vi "Test Bench v22 - TDMS.vi"() -> ()   [LabVIEW 2022 SP3]
doc: "Use this template to build a producer/consumer design pattern. Use this template when you need to execute a process, such as data analysis, when a data source, such as a triggered acquisition, produces data at an uneven rate and you need to execute the process when the data becomes available."
uses:
  WhiteNoise.ctl
  <vilib>/Utility/error.llb/DialogType.ctl
  <vilib>/Platform/TimedLoop/XDataNode/timing_clust.ctl
  <vilib>/Platform/TimedLoop/XDataNode/nitl_modes.ctl
  <vilib>/Platform/TimedLoop/XDataNode/wakeup.ctl
  <vilib>/DAQmx/write.llb/DAQmx Write (Analog Wfm 1Chan NSamp).vi
  <vilib>/DAQmx/read.llb/DAQmx Read (Analog Wfm 1Chan NSamp).vi
  <vilib>/DAQmx/miscellaneous.llb/DAQmx Fill In Error Info.vi
  <vilib>/measure/maspectr.llb/FFT Spectrum (Mag-Phase) for 1 Chan.vi
  <vilib>/platform/TimedLoop/XDataNode/XDataNode.xnode
  <vilib>/Platform/TimedLoop/XDataNode/XDNodeRunTimeDep.lvlib
  <vilib>/measure/NI_MAPro.lvlib
panel:
  out "SignalOut":waveform(dbl)(graph)
  out "FFT - Magnitude 2":cluster{"f0":dbl, "df":dbl, "magnitude":dbl[]}(graph)
  in  "view 2":T1={"dB On (F)"=FALSE, "unwrap phase (F)"=TRUE, "convert to degree (F)"=TRUE}
  out "FFT - Phase 2":cluster{"f0":dbl, "df":dbl, "phase":dbl[]}(graph)
  out "Accel":waveform(dbl)(graph)
  out "error out":errorcluster
  in  "stop":bool
  out "Iteration Duration 3":i64
  in  "samples per channel":i32=41200
  in  "Folder to save file to":path=path "C:/Users/LAV-UFSC-2023/Documents/LAV-TCC/Dados-Experimentos/Dados-Bancada-LABVIEW"
  out "# pending insert":i32
  out "# pending remove":i32
  out "# elements in queue":i32
  out "Processor 2":i32=-2
  out "Iteration Duration":i64
  out "Processor":i32=-2
  out "New file path":path
  in  "Log Data":bool=TRUE
  out "Iteration Duration 2":i64
  in  "Enable Output":bool=TRUE
  in  "Signal Output\nControl":enum32{"White Noise", "Harmonic"}(tab)
  in  "White Noise\nParameters":T3={"Seed"=0.0, "Standard Deviation"=2.0, "Reset"=FALSE, "Iterator"=1.0, "Lower Cut-Off"=5.0, "Upper Cut-Off"=350.0} {"Upper Cut-Off" min=5.0 max=350.0 step=10.0; "Lower Cut-Off" min=5.0 max=350.0 step=10.0; "Standard Deviation" min=0.001 max=3.0 step=0.05 format="%0.2p"}
  in  "Hamonic\nParameters":T4={"Waveform Type"=0, "Frequency (Hz)"=10.0, "Amplitude"=0.25} {"Frequency (Hz)" min=5.0 max=350.0 step=10.0 format="%0.2p"; "Waveform Type" items=["Sine Wave", "Triangle Wave", "Square Wave", "Sawtooth Wave"]; "Amplitude" min=0.001 max=0.3 step=0.05 format="%0.2p"}
  # "Debug Pannel"
  # "Filter"
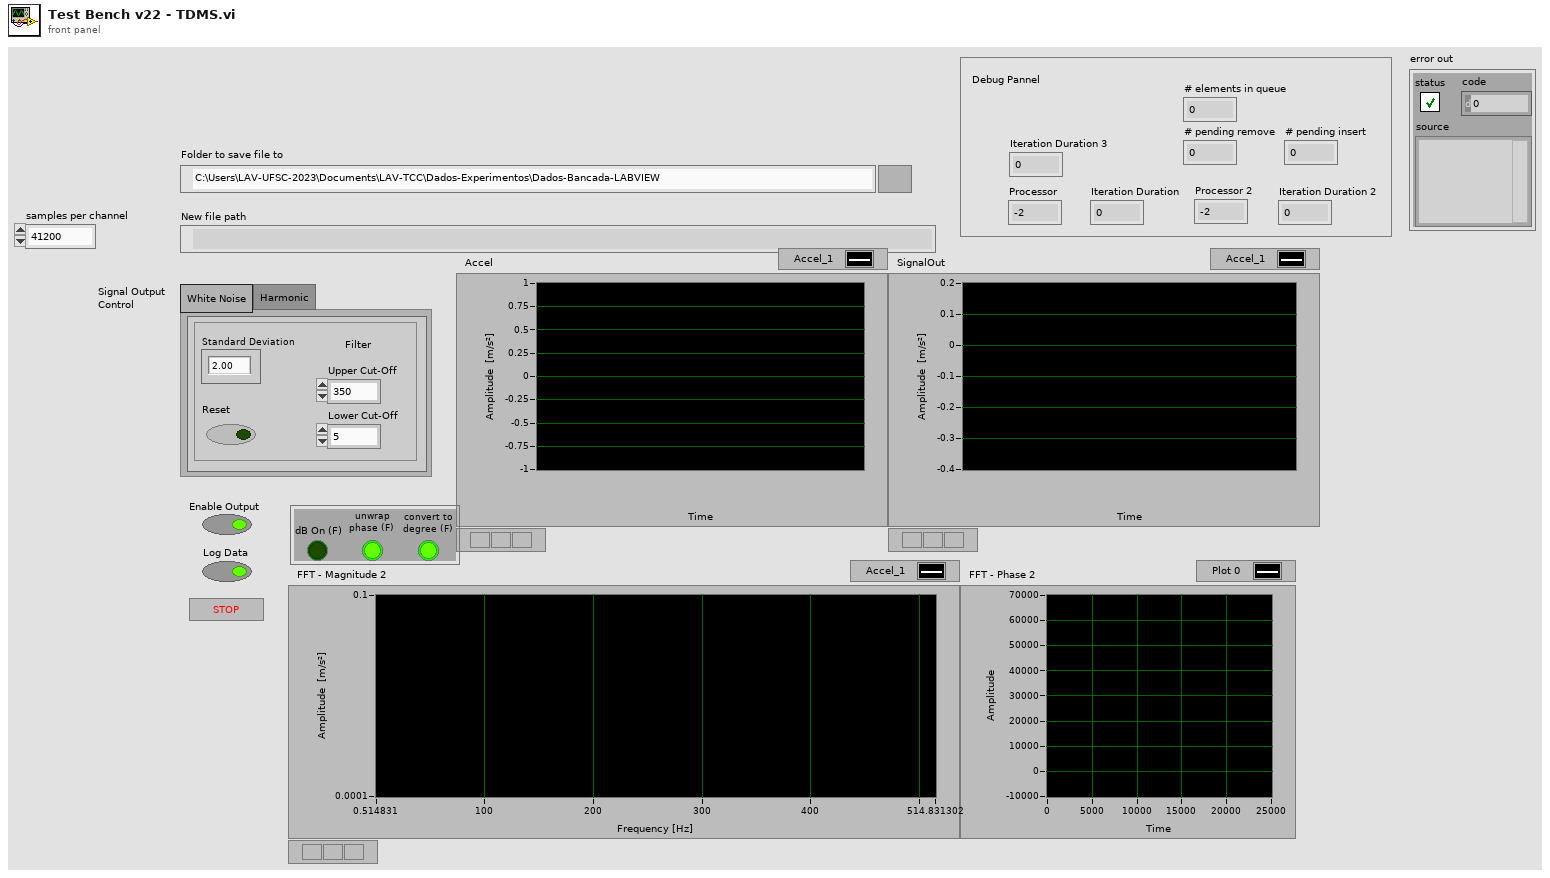
[diagram p1: front panel]
types:
  T1 = cluster{"dB On (F)":bool, "unwrap phase (F)":bool, "convert to degree (F)":bool}
  T2 = typedef "WhiteNoise.ctl" = dbl
  T3 = cluster{"Seed":T2, "Standard Deviation":dbl, "Reset":bool, "Iterator":dbl, "Lower Cut-Off":dbl, "Upper Cut-Off":dbl}
  T4 = cluster{"Waveform Type":u16, "Frequency (Hz)":dbl, "Amplitude":dbl}
  T5 = cluster{"FrameProperties":cluster{"Frame Duration":i64, "Actual Start [i]":i64}, "Data":waveform(dbl), "Identifier":enum16{"Accel", "SignalOut", "ButtonPress"}}
  T6 = typedef "XDNodeRunTimeDep.lvlib/timing_clust.ctl" = cluster{"Expected End [f-1]":u64, "Actual End [f-1]":u64, "Finished Late? [f-1]":bool, "Expected End [i-1]":u64, "Actual End [i-1]":u64, "Finished Late? [i-1]":bool, "Expected Start [i]":u64, "Actual Start [i]":u64, "Expected Start [f]":u64, "Actual Start [f]":u64, "Source Name":string, "Structure Name":string, "Period":i64, "Deadline":i64, "Offset":i64, "Start":i64, "Priority":i32, "Timeout":i32, "Mode":T7, "Wakeup Reason":T8, "Error":errorcluster, "Source Type":string, "Secondary Source Type":string, "Global End Time":u64, "Global Start Time":u64, "Frame Duration":u64, "Iteration Duration":u64, "Assigned CPU":i32, "I/O Scan Engine Mode":u32}
  T7 = typedef "XDNodeRunTimeDep.lvlib/nitl_modes.ctl" = enum32{"No Change", "Process missed periods, maintain original phase", "Discard missed periods, maintain original phase", "Process missed periods, ignore original phase", "Discard missed periods, ignore original phase"}
  T8 = typedef "XDNodeRunTimeDep.lvlib/wakeup.ctl" = enum32{"Normal", "Aborted", "Asynchronous wakeup", "Timing source error", "Timed loop error", "Timeout"}
  T9 = typedef "DialogType.ctl" = u16
  T10 = cluster{"Frame Duration":i64, "Actual Start [i]":i64}
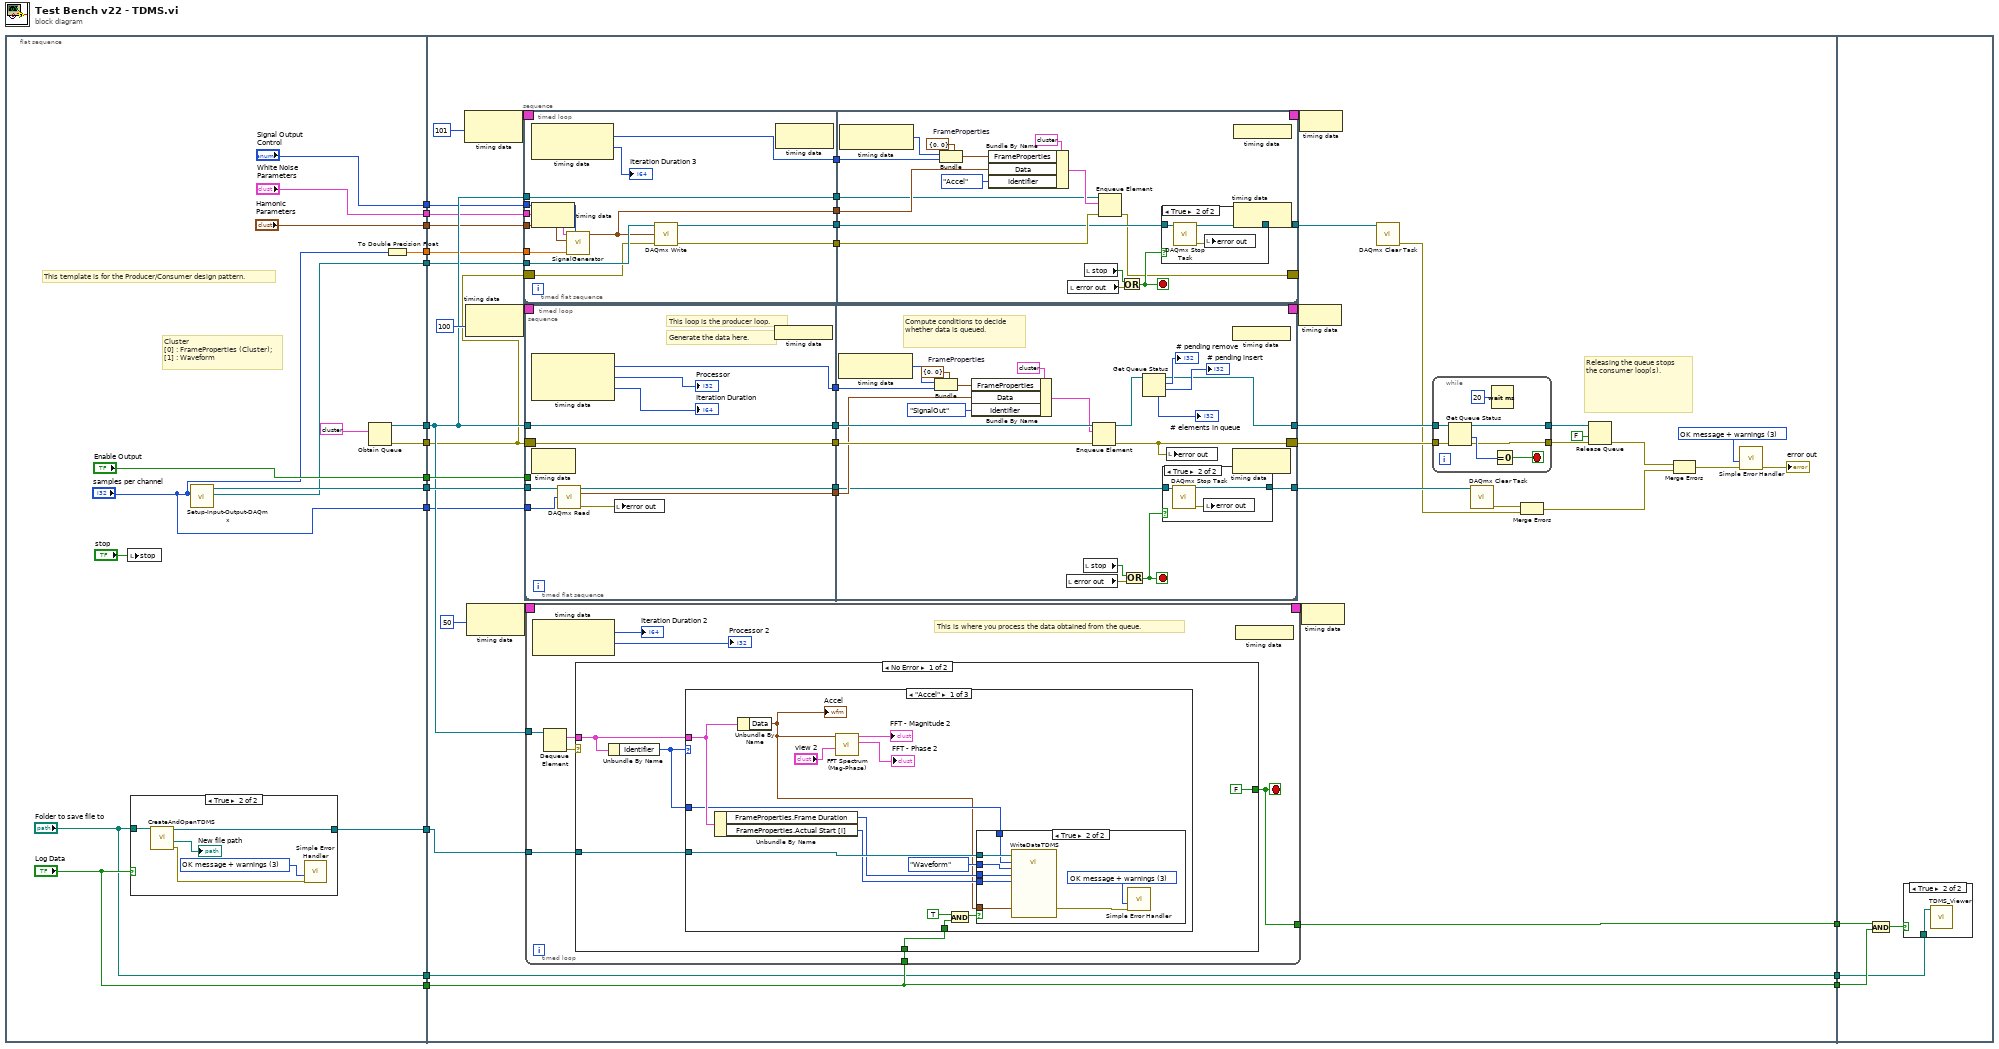
[diagram p0: block diagram]
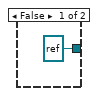
[diagram p2: hidden frame]
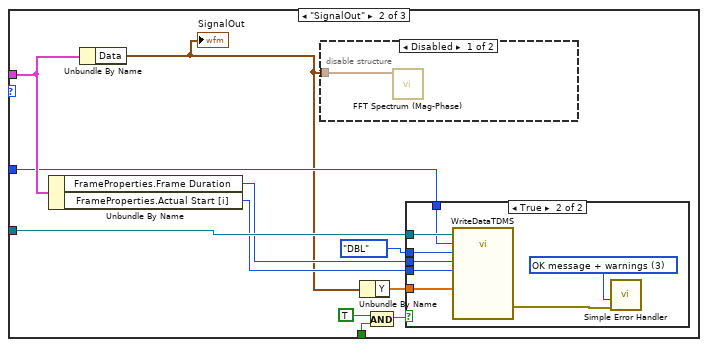
[diagram p5: hidden frame]
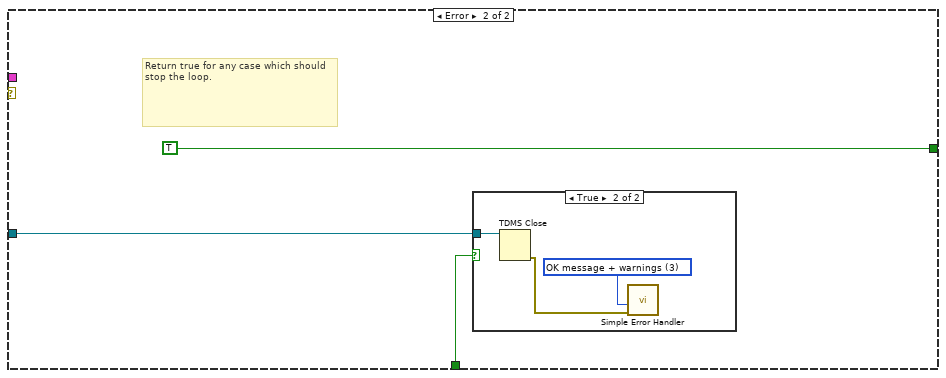
[diagram p9: hidden frame]
diagram:
  n1 = flat-sequence {
    tunnel: [w31] -> w16
    tunnel: [w30] -> w15
    tunnel: ["Log Data"] -> w14
    tunnel: ["Folder to save file to"] -> w10
    tunnel: ["Enable Output"] -> w9
    tunnel: [w25] -> w8
    tunnel: [w24] -> w7
    tunnel: ["samples per channel"] -> w6
    tunnel: [w23] -> w5
    tunnel: ["Signal Output\nControl"] -> w4
    tunnel: ["White Noise\nParameters"] -> w3
    tunnel: ["Hamonic\nParameters"] -> w2
    tunnel: [w19] -> w1
    tunnel: w16 -> [w69]
    tunnel: w15 -> [w66]
    tunnel: w14 -> [w64]
    tunnel: [w64] -> w13
    tunnel: [w63] -> w12
    tunnel: [w62] -> w11
    tunnel: w10 -> [w62]
    tunnel: w9 -> [w51]
    tunnel: w8 -> [w47]
    tunnel: w7 -> [w38]
    tunnel: w6 -> [w46]
    tunnel: w5 -> [w45]
    tunnel: w4 -> [w44]
    tunnel: w3 -> [w43]
    tunnel: w2 -> [w42]
    tunnel: w1 -> [w41]
    tunnel: w11 -> [w291]
    tunnel: w12 -> [w290]
    tunnel: w13 -> [w292]
    frame #0 {
      # "Cluster\n[0] : FrameProperties (Cluster);\n[1] : Waveform"
      # "This template is for the Producer/Consumer design pattern."
      n2 = local write "stop"("stop") -> ()
      n3 = case shown="True" "Log Data" {
        tunnel: [refnum<k34> refnum ("tdms file out") w34] -> w30
        tunnel: "Folder to save file to" -> [_ w33]
        frame False {
        }
        frame True {
          w36 = T9 3 items=["no dialog", "OK message", "continue or stop message", "OK message + warnings", "continue/stop + warnings"] ("type of dialog (OK msg:1)")
          n4 = call "CreateAndOpenTDMS.vi"("Folder to save file to"=w33) -> ("error out"=w37:errorcluster, "New file path"=→"New file path":path, "tdms file out"=w34:refnum<k34>)  [unwired: 8 in]
          n5 = call <vilib>:"Simple Error Handler.vi"("type of dialog (OK msg:1)"=w36, "error in (no error)"=w37) -> ()  [unwired: 3 in, 5 out]
        }
      }
      n6 = call "Setup-Input-Output-DAQmx.vi"("samples per channel"="samples per channel") -> ("Output task"=w23:refnum<k21>, "Input Task"=w31:refnum<k21>)  [unwired: 8 in, 1 out]
      n7 = Obtain Queue(element data type=T5 {"FrameProperties"={"Frame Duration"=0, "Actual Start [i]"=0}, "Data"={"t0"=timestamp(0 s since 1904-01-01), "dt"=1.0, "Y"=[]}, "Identifier"=enum."Accel"} ("input cluster")) -> (queue out=w25:refnum<queue>, error out=w24:errorcluster)  [unwired: 4 in, 1 out]
      n8 = To Double Precision Float(number="samples per channel") -> (double precision float=w19:dbl)
    }
    frame #1 {
      w53 = T9 3 items=["no dialog", "OK message", "continue or stop message", "OK message + warnings", "continue/stop + warnings"] ("type of dialog (OK msg:1)")
      # "Releasing the queue stops the consumer loop(s)."
      n9 = node-c288(101 ("Priority")) -> (w50:T6)
      n10 = node-c288(100 ("Priority")) -> (w74:T6)
      n11 = node-c288(50 ("Priority")) -> (w72:T6)
      n12 = timed-loop {
        timing: w50 -> [_]
        timing-out: [_] -> w49
        tunnel: w45 -> [w83]
        tunnel: w44 -> [w82]
        tunnel: w43 -> [w81]
        tunnel: w42 -> [w80]
        tunnel: w41 -> [w79]
        tunnel: [w78] -> w39
        shift-right: [w77] -> _
        shift-left: w38 -> [w76]
        tunnel: w47 -> [w75]
        stop <- w119 stop-if-true
        n13 = timed-sequence {
          timing: _ -> [_]
          timing-out: _ -> [_]
          tunnel: w83 -> [w97]
          tunnel: w82 -> [w96]
          tunnel: w81 -> [w95]
          tunnel: w80 -> [w94]
          tunnel: w79 -> [w90]
          tunnel: [w87] -> w78
          tunnel: [w86] -> w77
          tunnel: w76 -> [w85]
          tunnel: w75 -> [w84]
          n14 = timed-flat-sequence {
            tunnel: w97 -> [w109]
            tunnel: w96 -> [w108]
            tunnel: w95 -> [w107]
            tunnel: w94 -> [w106]
            tunnel: [w104] -> w93
            tunnel: [w103] -> w92
            tunnel: [w102] -> w91
            tunnel: w90 -> [w101]
            tunnel: [w100] -> w89
            tunnel: [w99] -> w88
            tunnel: w85 -> [w98]
            tunnel: w84 -> [w102]
            tunnel: w93 -> [w125]
            tunnel: w92 -> [w124]
            tunnel: w91 -> [w123]
            tunnel: w89 -> [w122]
            tunnel: w88 -> [w117]
            tunnel: [w118] -> w87
            tunnel: [w116] -> w86
            frame #0 {
              n15 = node-c288() -> (w104:i64, →"Iteration Duration 3":i64)  [unwired: 1 in]
              n16 = call "SignalGenerator.vi"("Signal Output\nControl"=w108, "#s"=w101, "Hamonic\nParameters"=w106, "White Noise\nParameters"=w107) -> ("Signal Out"=w103:waveform(dbl))  [unwired: 7 in]
              n17 = call-poly <vilib>:"DAQmx Write.vi"("task/channels in"=w109, "data"=w103, "error in"=w98) -> ("task out"=w99:refnum<k21>, "error out"=w100:errorcluster)  [unwired: 10 in, 1 out]
              n18 = node-c288() -> ()  [unwired: 1 in, 1 out]
            }
            frame #1 {
              w127 = T10 {"Frame Duration"=0, "Actual Start [i]"=0}  # FrameProperties
              n19 = node-c288() -> (w126:i64)  [unwired: 1 in]
              n20 = Bundle(cluster=w127, "Frame Duration"=w126, "Actual Start [i]"=w125) -> (w128:T10)
              n21 = Bundle By Name(cluster=T5 {"FrameProperties"={"Frame Duration"=0, "Actual Start [i]"=0}, "Data"={"t0"=timestamp(0 s since 1904-01-01), "dt"=1.0, "Y"=[]}, "Identifier"=enum."Accel"} ("input cluster"), "FrameProperties"=w128, "Data"=w124, "Identifier"=enum16{"Accel", "SignalOut", "ButtonPress"}."Accel") -> (w129:T5)
              n22 = local read "error out"() -> (w121:errorcluster)
              n23 = local read "stop"() -> (w120:bool)
              n24 = Enqueue Element(queue=w123, element=w129, error in (no error)=w122) -> (error out=w116:errorcluster)  [unwired: 1 in, 2 out]
              n25 = Or(x=w120, y=w121) -> (x .or. y?=w119:bool)
              n26 = case shown="True" w119 {
                tunnel: [w130 w133] -> w118
                tunnel: w117 -> [w130 w132]
                frame False {
                }
                frame True {
                  n27 = call <vilib>:"DAQmx Stop Task.vi"("task/channels in"=w132) -> ("task out"=w133:refnum<k21>, "error out"=w131:errorcluster)  [unwired: 13 in]
                  n28 = local write "error out"(w131) -> ()
                }
              }
              n29 = node-c288() -> ()  [unwired: 1 out]
            }
          }
        }
        n30 = node-c288() -> ()  [unwired: 1 in, 1 out]
        n31 = node-c288() -> ()  [unwired: 1 in, 1 out]
      }
      n32 = timed-loop {
        shift-right: [w224] -> w61
        shift-left: w38 -> [w226]
        tunnel: [w225] -> w68
        tunnel: w69 -> [w227]
        timing: w74 -> [_]
        timing-out: [_] -> w73
        tunnel: w51 -> [w223]
        tunnel: w46 -> [w222]
        tunnel: w47 -> [w221]
        tunnel: [w220] -> w65
        stop <- w258 stop-if-true
        n33 = timed-sequence {
          timing: _ -> [_]
          timing-out: _ -> [_]
          tunnel: w227 -> [w240]
          tunnel: w226 -> [w239]
          tunnel: [w233] -> w225
          tunnel: [w232] -> w224
          tunnel: w223 -> [w231]
          tunnel: w222 -> [w230]
          tunnel: w221 -> [w229]
          tunnel: [w228] -> w220
          n34 = timed-flat-sequence {
            tunnel: w240 -> [w244]
            tunnel: w239 -> [w250]
            tunnel: [w245] -> w238
            tunnel: [w250] -> w237
            tunnel: [w249] -> w236
            tunnel: [w248] -> w235
            tunnel: [w243] -> w234
            tunnel: w231 -> [_]
            tunnel: w230 -> [w242]
            tunnel: w229 -> [w249]
            tunnel: w238 -> [w263]
            tunnel: w237 -> [w276]
            tunnel: w236 -> [w275]
            tunnel: w235 -> [w273]
            tunnel: w234 -> [w272]
            tunnel: [w262] -> w233
            tunnel: [w261] -> w232
            tunnel: [w264] -> w228
            frame #0 {
              # "Generate the data here."
              # "This loop is the producer loop."
              n35 = node-c288() -> (w248:i64, →"Processor":i32, →"Iteration Duration":i64)  [unwired: 1 in]
              n36 = call-poly <vilib>:"DAQmx Read.vi"("task/channels in"=w244, "number of samples per channel"=w242) -> ("task out"=w245:refnum<k21>, "data"=w243:waveform(dbl), "error out"=w241:errorcluster)  [unwired: 11 in]
              n37 = local write "error out"(w241) -> ()
              n38 = node-c288() -> ()  [unwired: 1 out]
            }
            frame #1 {
              w269 = T10 {"Frame Duration"=0, "Actual Start [i]"=0}  # FrameProperties
              # "Compute conditions to decide whether data is queued."
              n39 = node-c288() -> (w274:i64)  [unwired: 1 in]
              n40 = Bundle(cluster=w269, "Frame Duration"=w274, "Actual Start [i]"=w273) -> (w270:T10)
              n41 = Bundle By Name(cluster=T5 {"FrameProperties"={"Frame Duration"=0, "Actual Start [i]"=0}, "Data"={"t0"=timestamp(0 s since 1904-01-01), "dt"=1.0, "Y"=[]}, "Identifier"=enum."Accel"} ("input cluster"), "FrameProperties"=w270, "Data"=w272, "Identifier"=enum16{"Accel", "SignalOut", "ButtonPress"}."SignalOut") -> (w271:T5)
              n42 = local read "error out"() -> (w260:errorcluster)
              n43 = local read "stop"() -> (w259:bool)
              n44 = Enqueue Element(queue=w275, element=w271, error in (no error)=w276) -> (queue out=w265:refnum<queue>, error out=w261:errorcluster)  [unwired: 1 in, 1 out]
              n45 = Or(x=w259, y=w260) -> (x .or. y?=w258:bool)
              n46 = Get Queue Status(queue=w265) -> (queue out=w264:refnum<queue>, # pending remove=→"# pending remove":i32, # pending insert=→"# pending insert":i32, # elements in queue=→"# elements in queue":i32)  [unwired: 2 in, 4 out]
              n47 = case shown="True" w258 {
                tunnel: [w277 w280] -> w262
                tunnel: w263 -> [w277 w279]
                frame False {
                }
                frame True {
                  n48 = call <vilib>:"DAQmx Stop Task.vi"("task/channels in"=w279) -> ("task out"=w280:refnum<k21>, "error out"=w278:errorcluster)  [unwired: 13 in]
                  n49 = local write "error out"(w278) -> ()
                }
              }
              n50 = local write "error out"(w261) -> ()
              n51 = node-c288() -> ()  [unwired: 1 out]
            }
          }
        }
        n52 = node-c288() -> ()  [unwired: 1 in, 1 out]
        n53 = node-c288() -> ()  [unwired: 1 in, 1 out]
      }
      n54 = timed-loop {
        tunnel: w47 -> [w157]
        timing: w72 -> [_]
        timing-out: [_] -> w71
        tunnel: w64 -> [w152]
        tunnel: [w150] -> w63
        tunnel: w66 -> [w153]
        stop <- w150 stop-if-true
        # "This is where you process the data obtained from the queue."
        n55 = node-c288() -> (→"Iteration Duration 2":i64, →"Processor 2":i32)  [unwired: 1 in]
        n56 = Dequeue Element(queue=w157) -> (element=w155:T5, error out=w156:errorcluster)  [unwired: 2 in, 2 out]
        n57 = case shown="No Error" w156 {
          tunnel: w155 -> [w163 _]
          tunnel: [FALSE TRUE] -> w150
          tunnel: w153 -> [w166 w210]
          tunnel: w152 -> [w164 w211]
          frame No Error {
            n58 = Unbundle By Name(w163) -> ("Identifier"=w162:enum16{"Accel", "SignalOut", "ButtonPress"})
            n59 = case shown="\"Accel\"" w162 {
              tunnel: w166 -> [w179 w198 _]
              tunnel: w164 -> [w178 w197 _]
              tunnel: w163 -> [w177 w196 _]
              tunnel: w162 -> [w169 w191 _]
              frame "Accel" {
                n60 = Unbundle By Name(w177) -> ("FrameProperties.Frame Duration"=w173:i64, "FrameProperties.Actual Start [i]"=w172:i64)
                n61 = Unbundle By Name(w177) -> ("Data"=w167:waveform(dbl))
                "Accel" <- w167
                n62 = call-poly <vilib>:"FFT Spectrum (Mag-Phase).vi"("view"="view 2", "time signal"=w167) -> ("phase"=→"FFT - Phase 2":cluster{"f0":dbl, "df":dbl, "phase":dbl[]}, "magnitude"=→"FFT - Magnitude 2":cluster{"f0":dbl, "df":dbl, "magnitude":dbl[]})  [unwired: 5 in, 3 out]
                n63 = And(x=TRUE, y=w178) -> (x .and. y?=w171:bool)
                n64 = case shown="True" w171 {
                  tunnel: w179 -> [_ w185]
                  tunnel: w173 -> [_ w184]
                  tunnel: w172 -> [_ w183]
                  tunnel: w169 -> [_ w182]
                  tunnel: enum16{"Waveform", "DBL"}."Waveform" ("InputDataType") -> [_ w181]
                  tunnel: w167 -> [_ w180]
                  frame False {
                  }
                  frame True {
                    w187 = T9 3 items=["no dialog", "OK message", "continue or stop message", "OK message + warnings", "continue/stop + warnings"] ("type of dialog (OK msg:1)")
                    n65 = call "WriteDataTDMS.vi"("Accel."=w180, "TDMS Input"=w185, "Identifier"=w182, "InputDataType"=w181, "TimeInterval"=w184, "ActualStart[f]"=w183) -> ("error out"=w186:errorcluster)  [unwired: 20 in, 1 out]
                    n66 = call <vilib>:"Simple Error Handler.vi"("type of dialog (OK msg:1)"=w187, "error in (no error)"=w186) -> ()  [unwired: 3 in, 5 out]
                  }
                }
              }
              frame "SignalOut" {
                n67 = Unbundle By Name(w196) -> ("FrameProperties.Frame Duration"=w195:i64, "FrameProperties.Actual Start [i]"=w194:i64)
                n68 = Unbundle By Name(w196) -> ("Data"=w190:waveform(dbl))
                "SignalOut" <- w190
                n69 = disable-structure shown="Disabled" {
                  disable-tunnel: w190 -> [w199 _]
                  frame Disabled {
                    n70 = call-poly <vilib>:"FFT Spectrum (Mag-Phase).vi"("time signal"=w199) -> ("phase"=w200:cluster{"f0":dbl, "df":dbl, "phase":dbl[]}, "magnitude"=w201:cluster{"f0":dbl, "df":dbl, "magnitude":dbl[]})  [unwired: 6 in, 3 out]
                  }
                  frame Enabled {
                  }
                }
                n71 = Unbundle By Name(w190) -> ("Y"=w189:dbl[])
                n72 = And(x=TRUE, y=w197) -> (x .and. y?=w193:bool)
                n73 = case shown="True" w193 {
                  tunnel: w198 -> [_ w207]
                  tunnel: w195 -> [_ w206]
                  tunnel: w194 -> [_ w205]
                  tunnel: w191 -> [_ w204]
                  tunnel: w189 -> [_ w203]
                  tunnel: enum16{"Waveform", "DBL"}."DBL" ("InputDataType") -> [_ w202]
                  frame False {
                  }
                  frame True {
                    w209 = T9 3 items=["no dialog", "OK message", "continue or stop message", "OK message + warnings", "continue/stop + warnings"] ("type of dialog (OK msg:1)")
                    n74 = call "WriteDataTDMS.vi"("TDMS Input"=w207, "Identifier"=w204, "InputDataType"=w202, "TimeInterval"=w206, "ActualStart[f]"=w205, "SignalOut"=w203) -> ("error out"=w208:errorcluster)  [unwired: 20 in, 1 out]
                    n75 = call <vilib>:"Simple Error Handler.vi"("type of dialog (OK msg:1)"=w209, "error in (no error)"=w208) -> ()  [unwired: 3 in, 5 out]
                  }
                }
              }
              frame "ButtonPress" {
              }
            }
          }
          frame Error {
            # "Return true for any case which should stop the loop."
            n76 = case shown="True" w211 {
              tunnel: w210 -> [_ w214]
              frame False {
              }
              frame True {
                w215 = T9 3 items=["no dialog", "OK message", "continue or stop message", "OK message + warnings", "continue/stop + warnings"] ("type of dialog (OK msg:1)")
                n77 = TDMS Close(11:w214) -> (0:w213:errorcluster)  [unwired: 1 in, 1 out]
                n78 = call <vilib>:"Simple Error Handler.vi"("type of dialog (OK msg:1)"=w215, "error in (no error)"=w213) -> ()  [unwired: 3 in, 5 out]
              }
            }
          }
        }
        n79 = node-c288() -> ()  [unwired: 1 out]
      }
      n80 = node-c288(w73) -> ()
      n81 = node-c288(w49) -> ()
      n82 = node-c288(w71) -> ()
      n83 = call <vilib>:"DAQmx Clear Task.vi"("task in"=w39) -> ("error out"=w57:errorcluster)  [unwired: 14 in]
      n84 = while {
        tunnel: w61 -> [w149]
        tunnel: w65 -> [w148]
        tunnel: [w145] -> w60
        tunnel: [w144] -> w59
        stop <- w146 stop-if-true
        n85 = Get Queue Status(queue=w148, error in (no error)=w149) -> (queue out=w144:refnum<queue>, # pending insert=w147:i32, error out=w145:errorcluster)  [unwired: 1 in, 5 out]
        n86 = Wait (ms)(milliseconds to wait=u32 20) -> ()  [unwired: 1 out]
        n87 = Equal To 0?(x=w147) -> (x = 0?=w146:bool)
      }
      n88 = call <vilib>:"DAQmx Clear Task.vi"("task in"=w68) -> ("error out"=w58:errorcluster)  [unwired: 14 in]
      n89 = Merge Errors(w58, w57) -> (w54:errorcluster)
      n90 = Release Queue(queue=w59, force destroy? (F)=FALSE, error in (no error)=w60) -> (error out=w55:errorcluster)  [unwired: 2 out]
      n91 = Merge Errors(w55, w54) -> (w56:errorcluster)
      n92 = call <vilib>:"Simple Error Handler.vi"("type of dialog (OK msg:1)"=w53, "error in (no error)"=w56) -> ("error out"=→"error out":errorcluster)  [unwired: 3 in, 4 out]
    }
    frame #2 {
      n93 = And(x=w290, y=w292) -> (x .and. y?=w293:bool)
      n94 = case shown="True" w293 {
        tunnel: w291 -> [_ w294]
        frame False {
        }
        frame True {
          n95 = call "TDMS_Viewer.vi"("Data Directory"=w294) -> ()  [unwired: 11 in]
        }
      }
    }
  }
